vi "BusB_Initialize Hardware References.vi"(8 "error in (no error)":errorcluster, 9 "HW Refnum in":string, 10 "BusB Baud Rate":string, 11 "BusB Visa Resource in":refnum<visa-resource-name>) -> (0 "error out":errorcluster, 2 "HW Refnum out":string, 3 "BusB Visa Resource out":refnum<visa-resource-name>)   [LabVIEW 2016, in "Impedance Data Acquisition and Decoding.lvlib"]
uses:
  Impedance Data Acquisition and Decoding.lvlib
  <vilib>/Instr/_visa.llb/VISA Configure Serial Port (Instr).vi
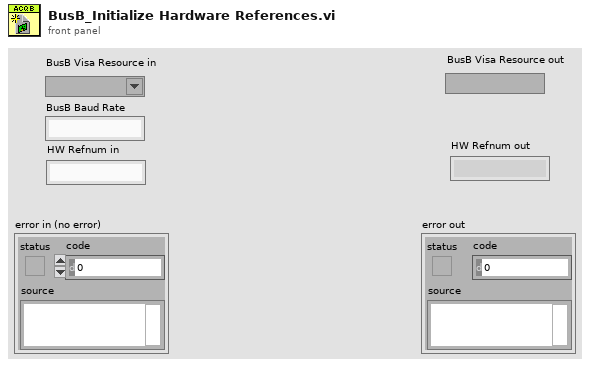
[diagram p1: front panel]
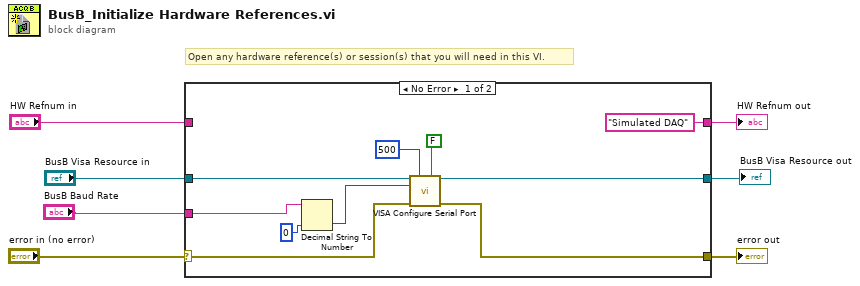
[diagram p0: block diagram]
diagram:
  # "Open any hardware reference(s) or session(s) that you will need in this VI."
  n1 = case shown="No Error" "error in (no error)" {
    selector: "error in (no error)" -> [w16 w19]
    tunnel: [w15 w19] -> w6
    tunnel: "HW Refnum in" -> [_ w20]
    tunnel: ["Simulated DAQ" ("HW Refnum in") w20] -> w4
    tunnel: [w14 w18] -> w3
    tunnel: "BusB Visa Resource in" -> [w13 w18]
    tunnel: "BusB Baud Rate" -> [w12 _]
    frame No Error {
      n2 = Decimal String To Number(string=w12, default (0L)=u32 0 ("default (0 I32)")) -> (number=w11:u32)  [unwired: 1 in, 1 out]
      n3 = call-poly "VISA Configure Serial Port"("VISA resource name"=w13, "timeout (10sec)"=u32 500, "Enable Termination\nChar (T)"=FALSE ("Enable Termination\nChar (T)"), "baud rate (9600)"=w11, "error in (no error)"=w16) -> ("VISA resource name out"=w14:refnum<visa-resource-name>, "error out"=w15:errorcluster)  [unwired: 9 in]
    }
    frame Error {
    }
  }
  "HW Refnum out" <- w4
  "error out" <- w6
  "BusB Visa Resource out" <- w3
